vi "command.vi"(0 "MoAgSy_GPG":refnum<class "MoAgSy_GPG.lvclass">, 1 "options file":path, 2 "keyringfile":path, 3 "Sec keyringfile":path, 4 "targetfile":path, 5 "sourcefile":path, 7 "error in (no error)":errorcluster, 8 "key-id":string, 9 "overwrite? (t)":bool=TRUE, 10 "Trust DB":path, 11 "reveiver":string[](array[string]), 12 "task":T1(ring), 13 "password":string) -> (15 "standard output":string, 16 "dup Trust DB":path, 17 "data error":bool, 19 "return code":i32, 20 "dup MoAgSy_GPG":refnum<class "MoAgSy_GPG.lvclass">, 21 "dup options file":path, 22 "dup keyringfile":path, 23 "dup Sec keyringfile":path, 24 "dup targetfile":path, 25 "dup sourcefile":path, 26 "standard error":string, 27 "error out":errorcluster)   [LabVIEW 2009, in "MoAgSy.lvlib" / "MoAgSy_GPG.lvclass"]
doc: "VI executes following gpg-commands (commandline):\nEncrypt\nDecrypt\nSign\nVerify\nSign&Encrypt\nVerify&Decrypt"
uses:
  MoAgSy_GPG.lvclass
  HGF_GPG/HGF_GPG.lvclass/HGF_GPG.lvclass
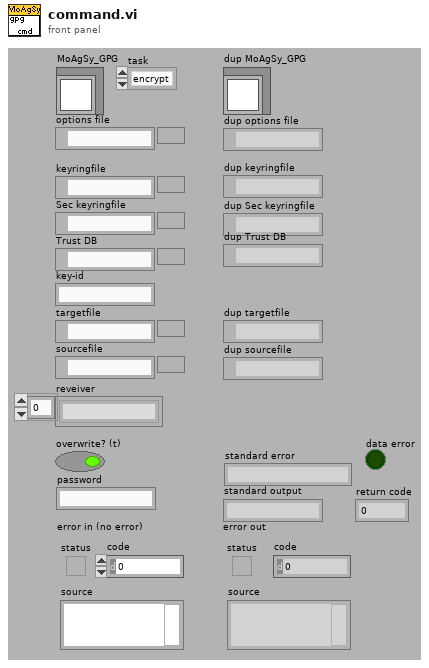
[diagram p1: front panel]
types:
  T1 = enum16{"encrypt", "decrypt", "sign", "verify", "sign & encrypt", "verify & decrypt"}
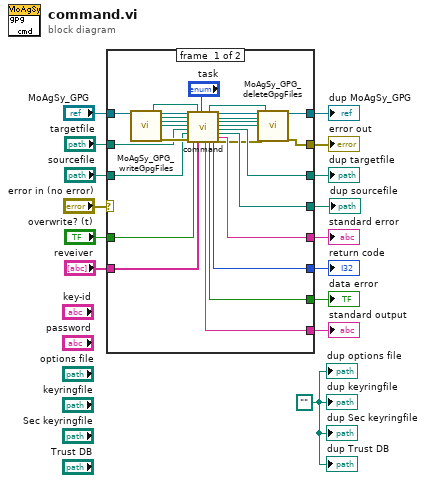
[diagram p0: block diagram]
diagram:
  w1 = path ""
  n1 = case shown="No Error" "error in (no error)" {
    selector: "error in (no error)" -> [_ w42]
    tunnel: "MoAgSy_GPG" -> [w29 w45]
    tunnel: "targetfile" -> [w40 w44]
    tunnel: "overwrite? (t)" -> [w39 _]
    tunnel: "reveiver" -> [w38 _]
    tunnel: [w36 _] -> w11
    tunnel: [w35 _] -> w10
    tunnel: [w34 _] -> w9
    tunnel: [w22 w45] -> w8
    tunnel: [w33 _] -> w7
    tunnel: [w20 w42] -> w6
    tunnel: [w32 w44] -> w5
    tunnel: "sourcefile" -> [w31 w43]
    tunnel: [w30 w43] -> w2
    frame #0 {
      n2 = call "MoAgSy_GPG_writeGpgFiles.vi"("MoAgSy_GPG"=w29) -> ("trust db file"=w24:path, "dup MoAgSy_GPG"=w28:refnum<class "MoAgSy_GPG.lvclass">, "options file"=w27:path, "keyring file"=w26:path, "sec keyring file"=w25:path, "error out"=w41:errorcluster)  [unwired: 1 in, 12 out]
      n3 = call-parent "command.vi"("HGF_GPG"=w28, "options file"=w27, "keyringfile"=w26, "Sec keyringfile"=w25, "targetfile"=w40, "sourcefile"=w31, "error in (no error)"=w41, "overwrite? (t)"=w39, "Trust DB"=w24, "reveiver"=w38, "task"="task") -> ("standard output"=w36:string, "dup Trust DB"=w19:path, "data error"=w35:bool, "return code"=w34:i32, "dup HGF_GPG"=w23:refnum<class "MoAgSy_GPG.lvclass">, "dup options file"=w18:path, "dup keyringfile"=w17:path, "dup Sec keyringfile"=w16:path, "dup targetfile"=w32:path, "dup sourcefile"=w30:path, "standard error"=w33:string, "error out"=w21:errorcluster)  [unwired: 2 in, 3 out]
      n4 = call "MoAgSy_GPG_deleteGpgFiles.vi"("MoAgSy_GPG"=w23, "options file"=w18, "keyringfile"=w17, "Sec keyringfile"=w16, "error in (no error)"=w21, "Trust DB"=w19) -> ("dup MoAgSy_GPG"=w22:refnum<class "MoAgSy_GPG.lvclass">, "error out"=w20:errorcluster)  [unwired: 12 out]
    }
    frame #1 {
    }
  }
  "error out" <- w6
  "dup MoAgSy_GPG" <- w8
  "dup targetfile" <- w5
  "dup sourcefile" <- w2
  "standard output" <- w11
  "standard error" <- w7
  "return code" <- w9
  "data error" <- w10
  "dup options file" <- w1
  "dup keyringfile" <- w1
  "dup Sec keyringfile" <- w1
  "dup Trust DB" <- w1
